vi "assignment - server.vi"() -> ()   [LabVIEW 2020]
panel:
  out "Automation":bool
  out "Vacation":bool
  out "DiningBrightness":u8
  out "KitchenBrightness":u8
  out "Bathroom2Brightness":u8
  out "Bathroom1Brightness":u8
  out "Laundry4Brightness":u8
  out "Laundry3Brightness":u8
  out "Laundry2Brightness":u8
  out "Laundry1Brightness":u8
  out "Bedroom2Brightness":u8
  out "Bedroom1Brightness":u8
  out "LivingRoomBrightness":u8
  out "DayCurtain":bool=TRUE
  out "NightTV":bool=TRUE
  out "Temperature Fluctuations":dbl(graph)
  in  "Upper Temp":dbl
  in  "Lower Temp":dbl
  out "Back Door  Open":bool
  out "Laundry 1 Open":bool
  out "Laundry 2 Open":bool
  out "Bathroom 2 Open":bool
  out "Laundry 4 Open":bool
  out "Bedroom 1 Open":bool
  out "Bedroom 2 Open":bool
  out "Front Door Open":bool
  out "Laundry 4 Close":bool
  out "Laundry 1 Close":bool
  out "Laundry 2 Close":bool
  out "Bathroom 2 Close":bool
  out "Bedroom 2 Close":bool
  out "Bedroom 1 Close":bool
  out "Back Door Close":bool
  out "Front Door Close":bool
  out "Thermometer":dbl(slide) scale=0.0..100.0
  out "Bedroom 2":dbl(slide) scale=0.0..1.0
  out "Bedroom 1":dbl(slide) scale=0.0..1.0
  in  "TV":refnum<k7>(container)
  out "Bathroom 2":bool
  out "Bathroom 1":bool
  out "Laundry 4":bool
  out "Laundry 3":bool
  out "Laundry 2":bool
  out "Laundry 1":bool
  out "Kitchen":bool
  out "Dining":bool
  out "Living Room":bool
  out "Bedroom 2":bool
  out "Bedroom 1":bool
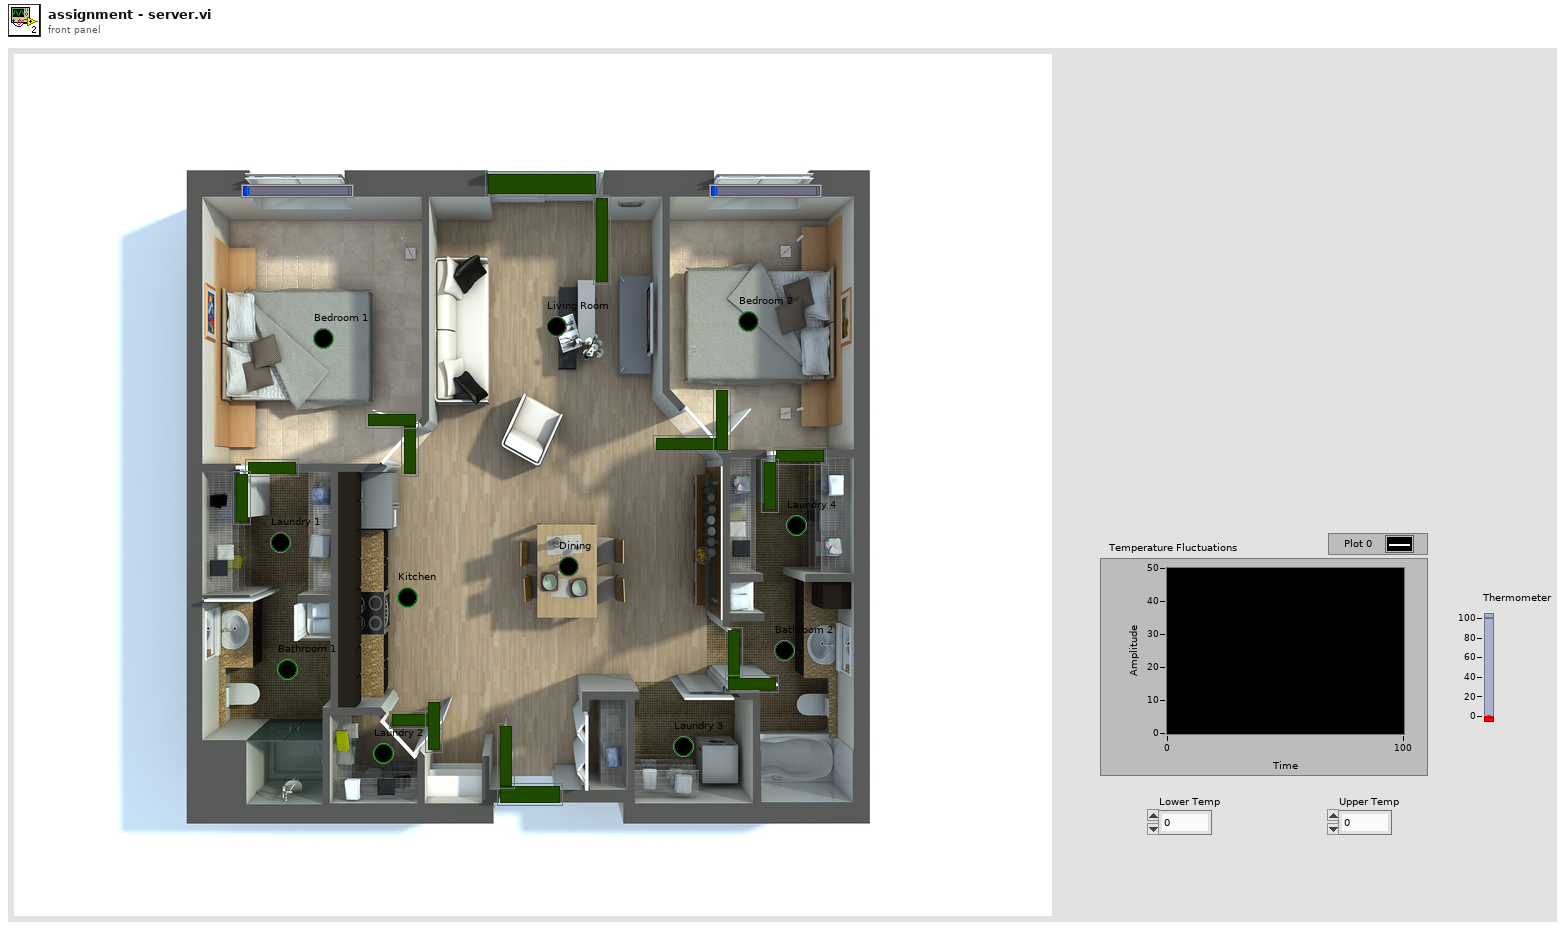
[diagram p1: front panel]
types:
  T1 = typedef "LVDateTimeRec.ctl" = cluster{"fractional second":dbl, "second":i32, "minute":i32, "hour":i32, "day of month":i32, "month":i32, "year":i32, "day of week":i32, "day of year":i32, "DST":i32}
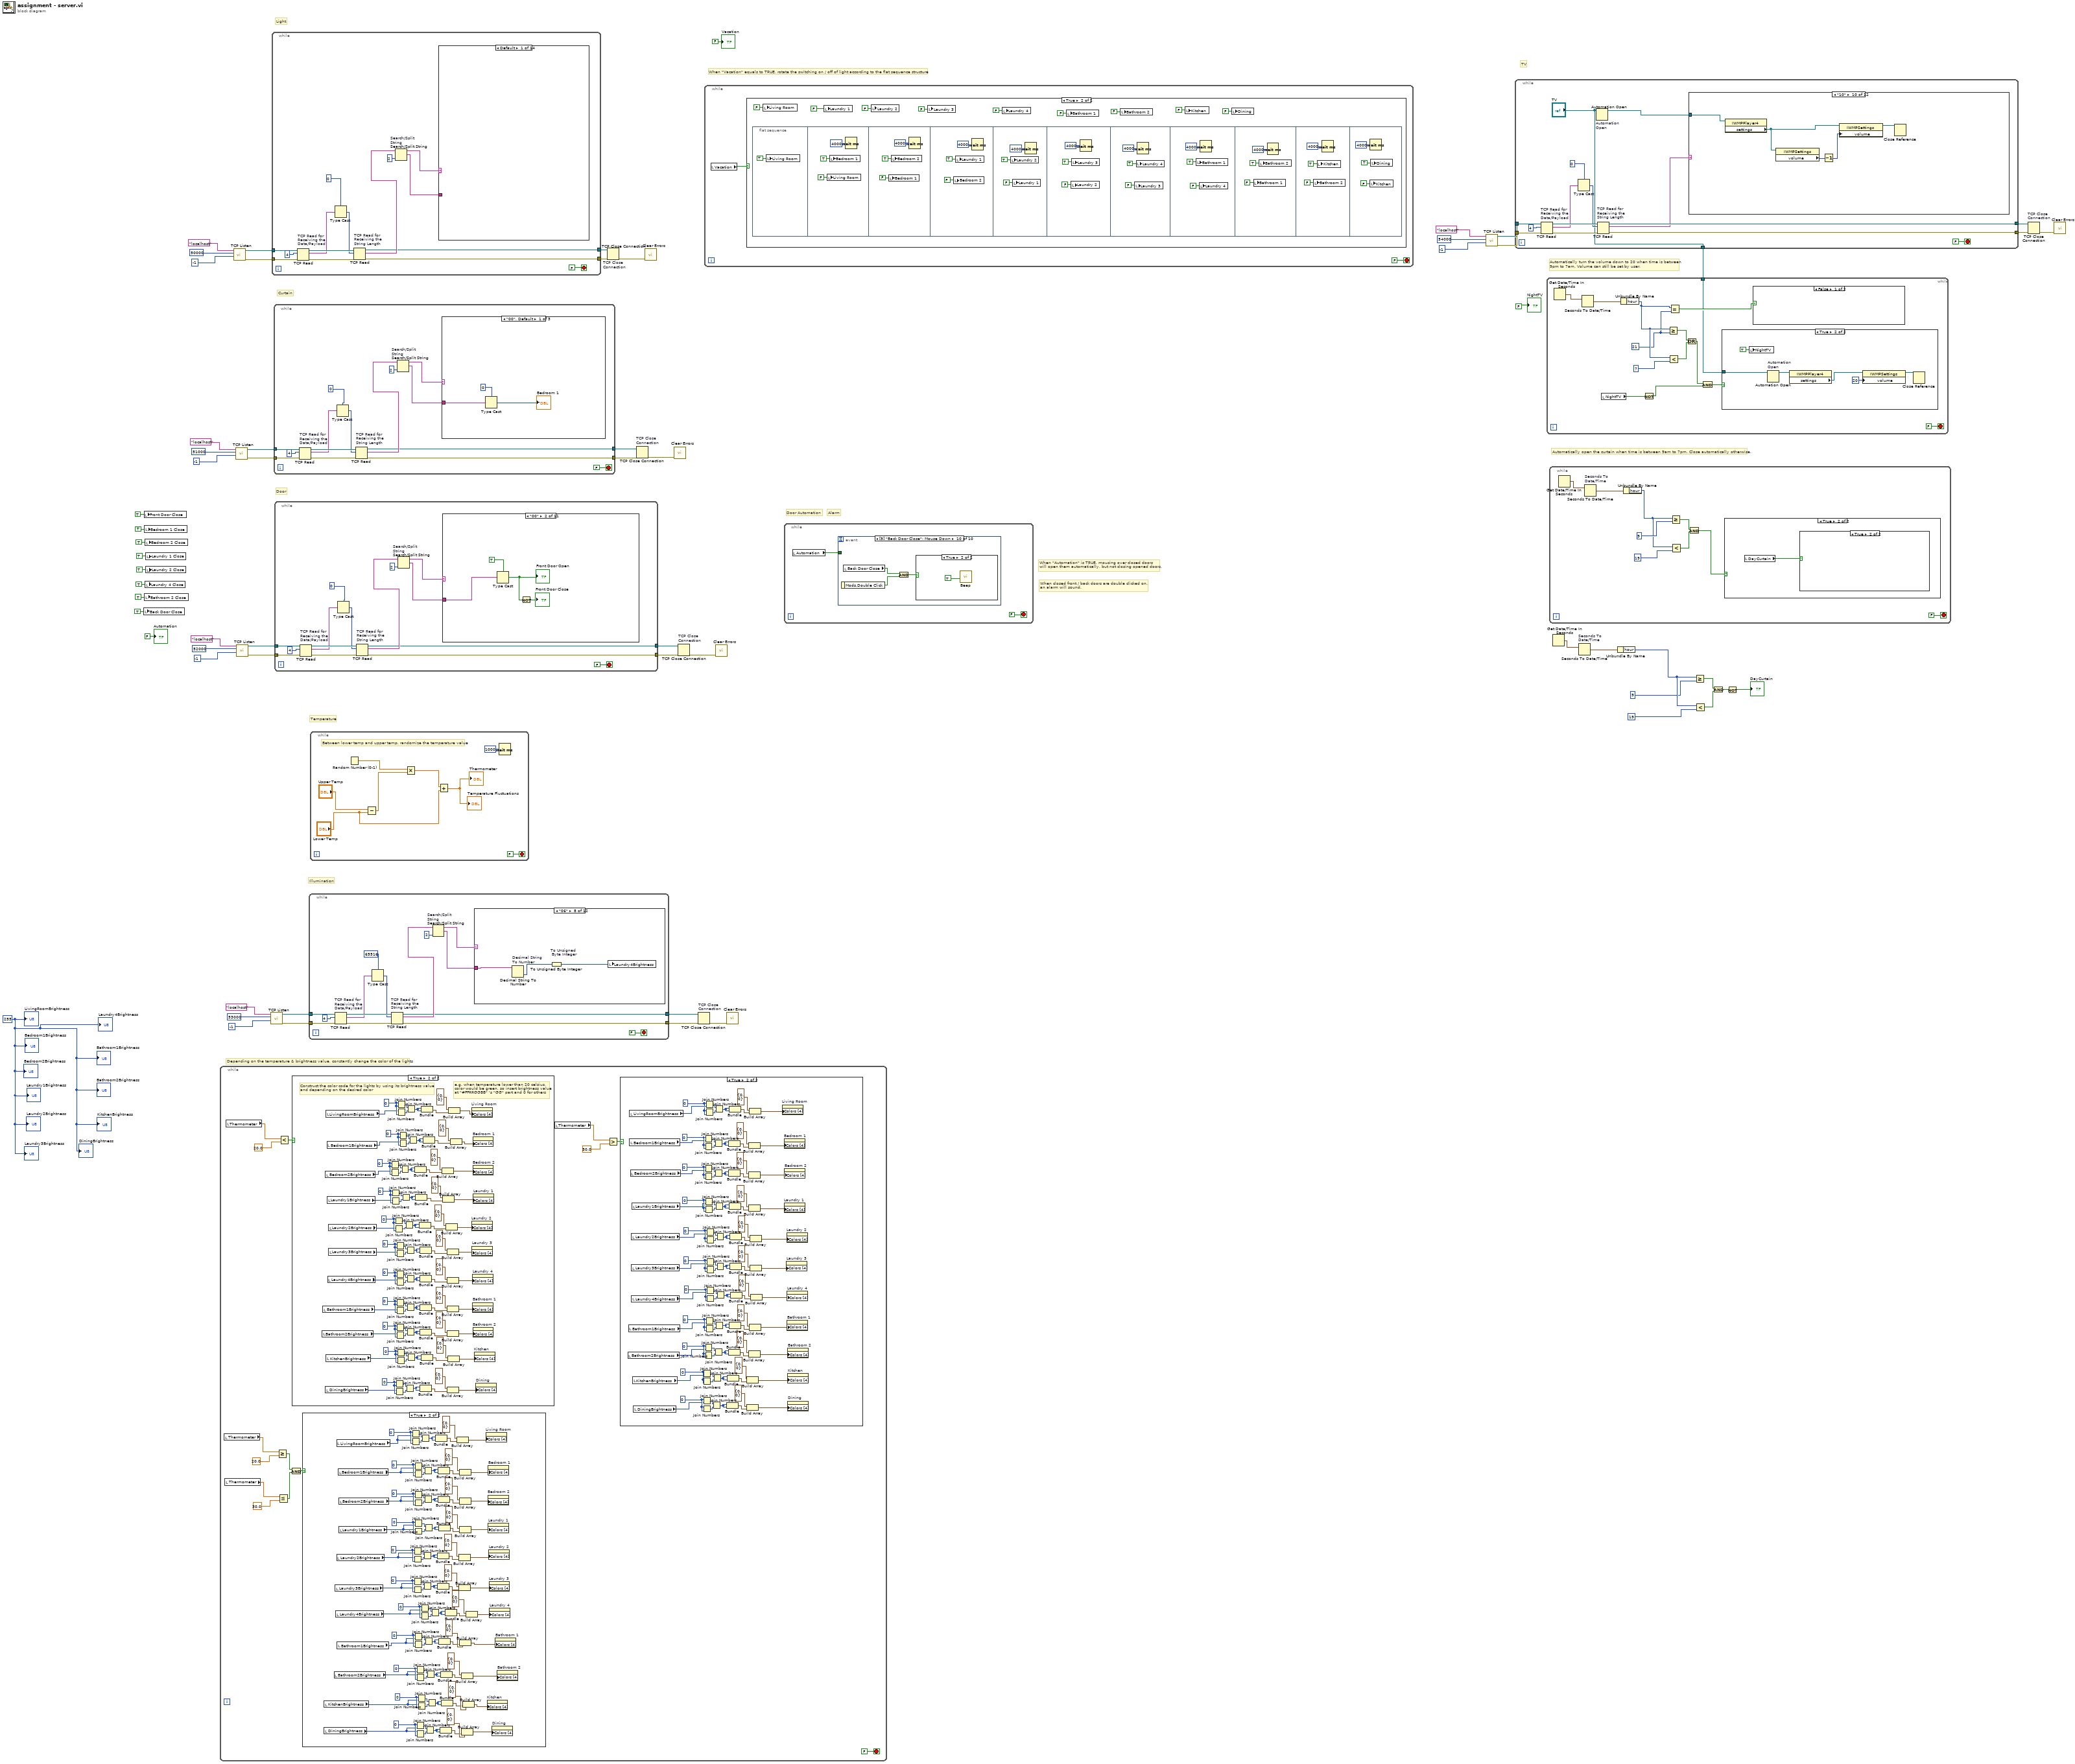
[diagram p0: block diagram]
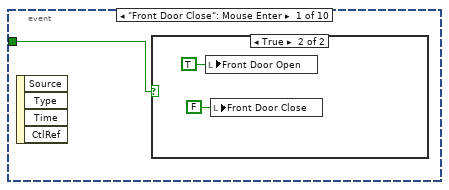
[diagram p2: hidden frame]
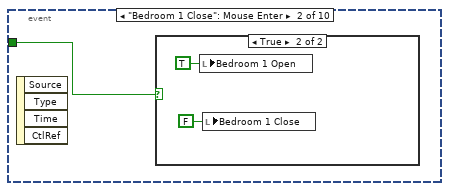
[diagram p4: hidden frame]
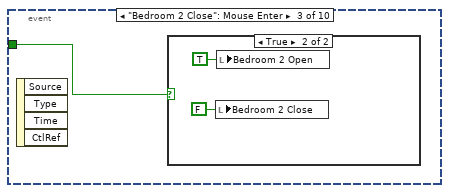
[diagram p6: hidden frame]
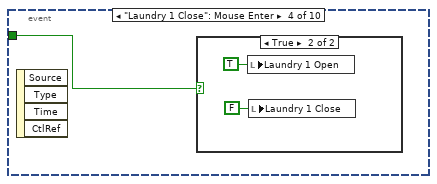
[diagram p8: hidden frame]
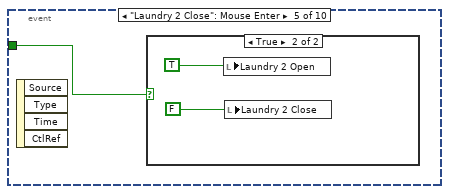
[diagram p10: hidden frame]
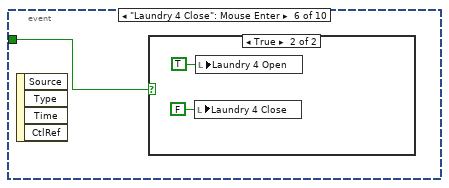
[diagram p12: hidden frame]
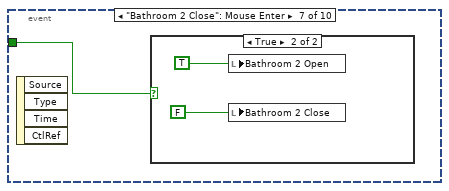
[diagram p14: hidden frame]
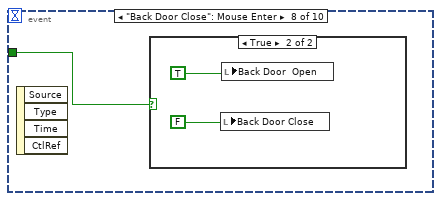
[diagram p16: hidden frame]
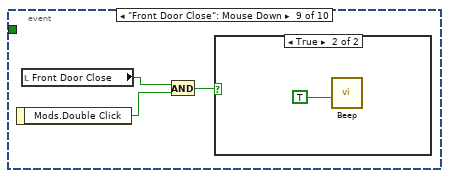
[diagram p18: hidden frame]
diagram:
  w3 = u8 255 ("LivingRoomBrightness")
  # "Automatically open the curtain when time is between 9am to 7pm. Close automatically otherwise."
  # "Automatically turn the volume down to 20 when time is between\n9pm to 7am. Volume can still be set by user."
  # "When \"Vacation\" equals to TRUE, rotate the switching on / off of light according to the flat sequence structure"
  # "When closed front / back doors are double clicked on,\nan alarm will sound."
  # "When \"Automation\" is TRUE, mousing over closed doors\nwill open them automatically, but not closing opened doors."
  # "Depending on the temperature & brightness value, constantly change the color of the lights"
  # "Alarm"
  # "Door Automation"
  # "Illumination"
  # "Temperature"
  # "Door"
  # "Curtain"
  # "TV"
  # "Light"
  n1 = local write "Back Door Close"(TRUE ("Back Door Close")) -> ()
  n2 = local write "Front Door Close"(TRUE ("Front Door Close")) -> ()
  n3 = local write "Bedroom 1 Close"(TRUE ("Bedroom 1 Close")) -> ()
  n4 = local write "Bathroom 2 Close"(TRUE ("Bathroom 2 Close")) -> ()
  n5 = local write "Bedroom 2 Close"(TRUE ("Bedroom 2 Close")) -> ()
  n6 = local write "Laundry 4 Close"(TRUE ("Laundry 4 Close")) -> ()
  n7 = local write "Laundry 1 Close"(TRUE ("Laundry 1 Close")) -> ()
  n8 = local write "Laundry 2 Close"(TRUE ("Laundry 2 Close")) -> ()
  n9 = while {
    stop <- FALSE stop-if-true
    n10 = local read "Thermometer"() -> (w68:dbl)
    n11 = local read "Thermometer"() -> (w65:dbl)
    n12 = local read "Thermometer"() -> (w76:dbl)
    n13 = Greater Or Equal?(x=w68, y=20.0) -> (x >= y?=w66:bool)
    n14 = Less Or Equal?(x=w65, y=30.0) -> (x <= y?=w63:bool)
    n15 = Less?(x=w76, y=20.0) -> (x < y?=w74:bool)
    n16 = And(x=w66, y=w63) -> (x .and. y?=w67:bool)
    n17 = case shown="True" w74 {
      frame False {
      }
      frame True {
        w256 = i8 0 ("hi")
        w264 = i8 0 ("hi")
        w272 = i8 0 ("hi")
        w280 = i8 0 ("hi")
        w288 = i8 0 ("hi")
        w296 = i8 0 ("hi")
        w304 = i8 0 ("hi")
        w312 = i8 0 ("hi")
        w320 = i8 0 ("hi")
        w328 = i8 0 ("hi")
        w335 = i8 0 ("hi")
        # "e.g. when temperature lower than 20 celsius,\ncolor would be green, so insert brightness value\nat \"#FFRRGGBB\" 's \"GG\" part and 0 for others"
        # "Construct the color code for the lights by using its brightness value\nand depending on the desired color"
        n18 = local read "Bathroom2Brightness"() -> (w270:u8)
        n19 = local read "Bathroom1Brightness"() -> (w278:u8)
        n20 = local read "Bedroom2Brightness"() -> (w318:u8)
        n21 = local read "DiningBrightness"() -> (w253:u8)
        n22 = local read "LivingRoomBrightness"() -> (w334:u8)
        n23 = local read "KitchenBrightness"() -> (w262:u8)
        n24 = local read "Bedroom1Brightness"() -> (w325:u8)
        n25 = local read "Laundry1Brightness"() -> (w310:u8)
        n26 = local read "Laundry4Brightness"() -> (w286:u8)
        n27 = local read "Laundry2Brightness"() -> (w302:u8)
        n28 = local read "Laundry3Brightness"() -> (w294:u8)
        n29 = Join Numbers(hi=w320, lo=w320) -> ((hi.lo)=w324:u16)
        n30 = Join Numbers(hi=w318, lo=w320) -> ((hi.lo)=w323:u16)
        n31 = Join Numbers(hi=w312, lo=w312) -> ((hi.lo)=w316:u16)
        n32 = Join Numbers(hi=w310, lo=w312) -> ((hi.lo)=w315:u16)
        n33 = Join Numbers(hi=w304, lo=w304) -> ((hi.lo)=w308:u16)
        n34 = Join Numbers(hi=w302, lo=w304) -> ((hi.lo)=w307:u16)
        n35 = Join Numbers(hi=w256, lo=w256) -> ((hi.lo)=w260:u16)
        n36 = Join Numbers(hi=w253, lo=w256) -> ((hi.lo)=w259:u16)
        n37 = Join Numbers(hi=w296, lo=w296) -> ((hi.lo)=w300:u16)
        n38 = Join Numbers(hi=w294, lo=w296) -> ((hi.lo)=w299:u16)
        n39 = Join Numbers(hi=w288, lo=w288) -> ((hi.lo)=w292:u16)
        n40 = Join Numbers(hi=w286, lo=w288) -> ((hi.lo)=w291:u16)
        n41 = Join Numbers(hi=w280, lo=w280) -> ((hi.lo)=w284:u16)
        n42 = Join Numbers(hi=w278, lo=w280) -> ((hi.lo)=w283:u16)
        n43 = Join Numbers(hi=w272, lo=w272) -> ((hi.lo)=w276:u16)
        n44 = Join Numbers(hi=w270, lo=w272) -> ((hi.lo)=w275:u16)
        n45 = Join Numbers(hi=w264, lo=w264) -> ((hi.lo)=w268:u16)
        n46 = Join Numbers(hi=w262, lo=w264) -> ((hi.lo)=w267:u16)
        n47 = Join Numbers(hi=w335, lo=w335) -> ((hi.lo)=w340:u16)
        n48 = Join Numbers(hi=w334, lo=w335) -> ((hi.lo)=w339:u16)
        n49 = Join Numbers(hi=w328, lo=w328) -> ((hi.lo)=w332:u16)
        n50 = Join Numbers(hi=w325, lo=w328) -> ((hi.lo)=w331:u16)
        n51 = Join Numbers(hi=w324, lo=w323) -> ((hi.lo)=w322:u32)
        n52 = Join Numbers(hi=w316, lo=w315) -> ((hi.lo)=w314:u32)
        n53 = Join Numbers(hi=w308, lo=w307) -> ((hi.lo)=w306:u32)
        n54 = Join Numbers(hi=w260, lo=w259) -> ((hi.lo)=w258:u32)
        n55 = Join Numbers(hi=w300, lo=w299) -> ((hi.lo)=w298:u32)
        n56 = Join Numbers(hi=w292, lo=w291) -> ((hi.lo)=w290:u32)
        n57 = Join Numbers(hi=w284, lo=w283) -> ((hi.lo)=w282:u32)
        n58 = Join Numbers(hi=w276, lo=w275) -> ((hi.lo)=w274:u32)
        n59 = Join Numbers(hi=w268, lo=w267) -> ((hi.lo)=w266:u32)
        n60 = Join Numbers(hi=w340, lo=w339) -> ((hi.lo)=w338:u32)
        n61 = Join Numbers(hi=w332, lo=w331) -> ((hi.lo)=w330:u32)
        n62 = Bundle "Bundle"(w322, w322) -> (w321:cluster{u32, u32})  [unwired: 1 in]
        n63 = Bundle "Bundle"(w314, w314) -> (w313:cluster{u32, u32})  [unwired: 1 in]
        n64 = Bundle "Bundle"(w306, w306) -> (w305:cluster{u32, u32})  [unwired: 1 in]
        n65 = Bundle "Bundle"(w258, w258) -> (w257:cluster{u32, u32})  [unwired: 1 in]
        n66 = Bundle "Bundle"(w298, w298) -> (w297:cluster{u32, u32})  [unwired: 1 in]
        n67 = Bundle "Bundle"(w290, w290) -> (w289:cluster{u32, u32})  [unwired: 1 in]
        n68 = Bundle "Bundle"(w282, w282) -> (w281:cluster{u32, u32})  [unwired: 1 in]
        n69 = Bundle "Bundle"(w274, w274) -> (w273:cluster{u32, u32})  [unwired: 1 in]
        n70 = Bundle "Bundle"(w266, w266) -> (w265:cluster{u32, u32})  [unwired: 1 in]
        n71 = Bundle "Bundle"(w338, w338) -> (w337:cluster{u32, u32})  [unwired: 1 in]
        n72 = Bundle "Bundle"(w330, w330) -> (w329:cluster{u32, u32})  [unwired: 1 in]
        n73 = Build Array "Build Array"(cluster{u32, u32} {0, 0} ("element"), w321) -> (w317:cluster{u32, u32}[])
        n74 = Build Array "Build Array"(cluster{u32, u32} {0, 0} ("element"), w313) -> (w309:cluster{u32, u32}[])
        n75 = Build Array "Build Array"(cluster{u32, u32} {0, 0} ("element"), w305) -> (w301:cluster{u32, u32}[])
        n76 = Build Array "Build Array"(cluster{u32, u32} {0, 0} ("element"), w257) -> (w254:cluster{u32, u32}[])
        n77 = Build Array "Build Array"(cluster{u32, u32} {0, 0} ("element"), w297) -> (w293:cluster{u32, u32}[])
        n78 = Build Array "Build Array"(cluster{u32, u32} {0, 0} ("element"), w289) -> (w285:cluster{u32, u32}[])
        n79 = Build Array "Build Array"(cluster{u32, u32} {0, 0} ("element"), w281) -> (w277:cluster{u32, u32}[])
        n80 = Build Array "Build Array"(cluster{u32, u32} {0, 0} ("element"), w273) -> (w269:cluster{u32, u32}[])
        n81 = Build Array "Build Array"(cluster{u32, u32} {0, 0} ("element"), w265) -> (w261:cluster{u32, u32}[])
        n82 = Build Array "Build Array"(cluster{u32, u32} {0, 0} ("element"), w337) -> (w336:cluster{u32, u32}[])
        n83 = Build Array "Build Array"(cluster{u32, u32} {0, 0} ("element"), w329) -> (w326:cluster{u32, u32}[])
        n84 = property on="Living Room" class="Bool (strict)"("Colors [4]"=w336) -> ()  [unwired: 2 in, 2 out]
        n85 = property on="Laundry 2" class="Bool (strict)"("Colors [4]"=w301) -> ()  [unwired: 2 in, 2 out]
        n86 = property on="Laundry 3" class="Bool (strict)"("Colors [4]"=w293) -> ()  [unwired: 2 in, 2 out]
        n87 = property on="Laundry 4" class="Bool (strict)"("Colors [4]"=w285) -> ()  [unwired: 2 in, 2 out]
        n88 = property on="Bathroom 1" class="Bool (strict)"("Colors [4]"=w277) -> ()  [unwired: 2 in, 2 out]
        n89 = property on="Bedroom 1" class="Bool (strict)"("Colors [4]"=w326) -> ()  [unwired: 2 in, 2 out]
        n90 = property on="Bedroom 2" class="Bool (strict)"("Colors [4]"=w317) -> ()  [unwired: 2 in, 2 out]
        n91 = property on="Bathroom 2" class="Bool (strict)"("Colors [4]"=w269) -> ()  [unwired: 2 in, 2 out]
        n92 = property on="Laundry 1" class="Bool (strict)"("Colors [4]"=w309) -> ()  [unwired: 2 in, 2 out]
        n93 = property on="Kitchen" class="Bool (strict)"("Colors [4]"=w261) -> ()  [unwired: 2 in, 2 out]
        n94 = property on="Dining" class="Bool (strict)"("Colors [4]"=w254) -> ()  [unwired: 2 in, 2 out]
      }
    }
    n95 = case shown="True" w67 {
      frame False {
      }
      frame True {
        w82 = i8 0 ("hi")
        w90 = i8 0 ("hi")
        w98 = i8 0 ("hi")
        w106 = i8 0 ("hi")
        w114 = i8 0 ("hi")
        w122 = i8 0 ("hi")
        w130 = i8 0 ("hi")
        w138 = i8 0 ("hi")
        w146 = i8 0 ("hi")
        w154 = i8 0 ("hi")
        w161 = i8 0 ("hi")
        n96 = local read "KitchenBrightness"() -> (w86:u8)
        n97 = local read "DiningBrightness"() -> (w78:u8)
        n98 = local read "Bathroom2Brightness"() -> (w94:u8)
        n99 = local read "Laundry3Brightness"() -> (w118:u8)
        n100 = local read "Laundry4Brightness"() -> (w110:u8)
        n101 = local read "LivingRoomBrightness"() -> (w160:u8)
        n102 = local read "Laundry2Brightness"() -> (w126:u8)
        n103 = local read "Bathroom1Brightness"() -> (w102:u8)
        n104 = local read "Bedroom1Brightness"() -> (w150:u8)
        n105 = local read "Bedroom2Brightness"() -> (w142:u8)
        n106 = local read "Laundry1Brightness"() -> (w134:u8)
        n107 = Join Numbers(hi=w161, lo=w160) -> ((hi.lo)=w162:u16)
        n108 = Join Numbers(hi=w160, lo=w161) -> ((hi.lo)=w163:u16)
        n109 = Join Numbers(hi=w130, lo=w126) -> ((hi.lo)=w129:u16)
        n110 = Join Numbers(hi=w126, lo=w130) -> ((hi.lo)=w128:u16)
        n111 = Join Numbers(hi=w122, lo=w118) -> ((hi.lo)=w121:u16)
        n112 = Join Numbers(hi=w118, lo=w122) -> ((hi.lo)=w120:u16)
        n113 = Join Numbers(hi=w154, lo=w150) -> ((hi.lo)=w153:u16)
        n114 = Join Numbers(hi=w150, lo=w154) -> ((hi.lo)=w152:u16)
        n115 = Join Numbers(hi=w146, lo=w142) -> ((hi.lo)=w145:u16)
        n116 = Join Numbers(hi=w142, lo=w146) -> ((hi.lo)=w144:u16)
        n117 = Join Numbers(hi=w138, lo=w134) -> ((hi.lo)=w137:u16)
        n118 = Join Numbers(hi=w134, lo=w138) -> ((hi.lo)=w136:u16)
        n119 = Join Numbers(hi=w106, lo=w102) -> ((hi.lo)=w105:u16)
        n120 = Join Numbers(hi=w102, lo=w106) -> ((hi.lo)=w104:u16)
        n121 = Join Numbers(hi=w82, lo=w78) -> ((hi.lo)=w81:u16)
        n122 = Join Numbers(hi=w78, lo=w82) -> ((hi.lo)=w80:u16)
        n123 = Join Numbers(hi=w98, lo=w94) -> ((hi.lo)=w97:u16)
        n124 = Join Numbers(hi=w94, lo=w98) -> ((hi.lo)=w96:u16)
        n125 = Join Numbers(hi=w90, lo=w86) -> ((hi.lo)=w89:u16)
        n126 = Join Numbers(hi=w86, lo=w90) -> ((hi.lo)=w88:u16)
        n127 = Join Numbers(hi=w114, lo=w110) -> ((hi.lo)=w113:u16)
        n128 = Join Numbers(hi=w110, lo=w114) -> ((hi.lo)=w112:u16)
        n129 = Join Numbers(hi=w162, lo=w163) -> ((hi.lo)=w164:u32)
        n130 = Join Numbers(hi=w129, lo=w128) -> ((hi.lo)=w127:u32)
        n131 = Join Numbers(hi=w121, lo=w120) -> ((hi.lo)=w119:u32)
        n132 = Join Numbers(hi=w153, lo=w152) -> ((hi.lo)=w151:u32)
        n133 = Join Numbers(hi=w145, lo=w144) -> ((hi.lo)=w143:u32)
        n134 = Join Numbers(hi=w137, lo=w136) -> ((hi.lo)=w135:u32)
        n135 = Join Numbers(hi=w105, lo=w104) -> ((hi.lo)=w103:u32)
        n136 = Join Numbers(hi=w81, lo=w80) -> ((hi.lo)=w79:u32)
        n137 = Join Numbers(hi=w97, lo=w96) -> ((hi.lo)=w95:u32)
        n138 = Join Numbers(hi=w89, lo=w88) -> ((hi.lo)=w87:u32)
        n139 = Join Numbers(hi=w113, lo=w112) -> ((hi.lo)=w111:u32)
        n140 = Bundle(w164, w164) -> (w159:cluster{u32, u32})  [unwired: 1 in]
        n141 = Bundle(w127, w127) -> (w131:cluster{u32, u32})  [unwired: 1 in]
        n142 = Bundle(w119, w119) -> (w123:cluster{u32, u32})  [unwired: 1 in]
        n143 = Bundle(w151, w151) -> (w155:cluster{u32, u32})  [unwired: 1 in]
        n144 = Bundle(w143, w143) -> (w147:cluster{u32, u32})  [unwired: 1 in]
        n145 = Bundle(w135, w135) -> (w139:cluster{u32, u32})  [unwired: 1 in]
        n146 = Bundle(w103, w103) -> (w107:cluster{u32, u32})  [unwired: 1 in]
        n147 = Bundle(w79, w79) -> (w83:cluster{u32, u32})  [unwired: 1 in]
        n148 = Bundle(w95, w95) -> (w99:cluster{u32, u32})  [unwired: 1 in]
        n149 = Bundle(w87, w87) -> (w91:cluster{u32, u32})  [unwired: 1 in]
        n150 = Bundle(w111, w111) -> (w115:cluster{u32, u32})  [unwired: 1 in]
        n151 = Build Array "Build Array"(cluster{u32, u32} {0, 0} ("element"), w159) -> (w157:cluster{u32, u32}[])
        n152 = Build Array "Build Array"(cluster{u32, u32} {0, 0} ("element"), w131) -> (w125:cluster{u32, u32}[])
        n153 = Build Array "Build Array"(cluster{u32, u32} {0, 0} ("element"), w123) -> (w117:cluster{u32, u32}[])
        n154 = Build Array "Build Array"(cluster{u32, u32} {0, 0} ("element"), w155) -> (w149:cluster{u32, u32}[])
        n155 = Build Array "Build Array"(cluster{u32, u32} {0, 0} ("element"), w147) -> (w141:cluster{u32, u32}[])
        n156 = Build Array "Build Array"(cluster{u32, u32} {0, 0} ("element"), w139) -> (w133:cluster{u32, u32}[])
        n157 = Build Array "Build Array"(cluster{u32, u32} {0, 0} ("element"), w107) -> (w101:cluster{u32, u32}[])
        n158 = Build Array "Build Array"(cluster{u32, u32} {0, 0} ("element"), w83) -> (w77:cluster{u32, u32}[])
        n159 = Build Array "Build Array"(cluster{u32, u32} {0, 0} ("element"), w99) -> (w93:cluster{u32, u32}[])
        n160 = Build Array "Build Array"(cluster{u32, u32} {0, 0} ("element"), w91) -> (w85:cluster{u32, u32}[])
        n161 = Build Array "Build Array"(cluster{u32, u32} {0, 0} ("element"), w115) -> (w109:cluster{u32, u32}[])
        n162 = property on="Living Room" class="Bool (strict)"("Colors [4]"=w157) -> ()  [unwired: 2 in, 2 out]
        n163 = property on="Kitchen" class="Bool (strict)"("Colors [4]"=w85) -> ()  [unwired: 2 in, 2 out]
        n164 = property on="Bedroom 2" class="Bool (strict)"("Colors [4]"=w141) -> ()  [unwired: 2 in, 2 out]
        n165 = property on="Bedroom 1" class="Bool (strict)"("Colors [4]"=w149) -> ()  [unwired: 2 in, 2 out]
        n166 = property on="Laundry 1" class="Bool (strict)"("Colors [4]"=w133) -> ()  [unwired: 2 in, 2 out]
        n167 = property on="Laundry 2" class="Bool (strict)"("Colors [4]"=w125) -> ()  [unwired: 2 in, 2 out]
        n168 = property on="Laundry 3" class="Bool (strict)"("Colors [4]"=w117) -> ()  [unwired: 2 in, 2 out]
        n169 = property on="Laundry 4" class="Bool (strict)"("Colors [4]"=w109) -> ()  [unwired: 2 in, 2 out]
        n170 = property on="Dining" class="Bool (strict)"("Colors [4]"=w77) -> ()  [unwired: 2 in, 2 out]
        n171 = property on="Bathroom 1" class="Bool (strict)"("Colors [4]"=w101) -> ()  [unwired: 2 in, 2 out]
        n172 = property on="Bathroom 2" class="Bool (strict)"("Colors [4]"=w93) -> ()  [unwired: 2 in, 2 out]
      }
    }
    n173 = local read "Thermometer"() -> (w70:dbl)
    n174 = Greater?(x=w70, y=30.0) -> (0:w72:bool)
    n175 = case shown="True" w72 {
      frame False {
      }
      frame True {
        w169 = i8 0 ("hi")
        w176 = i8 0 ("hi")
        w185 = i8 0 ("hi")
        w193 = i8 0 ("hi")
        w201 = i8 0 ("hi")
        w209 = i8 0 ("hi")
        w216 = i8 0 ("hi")
        w225 = i8 0 ("hi")
        w233 = i8 0 ("hi")
        w241 = i8 0 ("hi")
        w248 = i8 0 ("hi")
        n176 = local read "Bathroom2Brightness"() -> (w182:u8)
        n177 = local read "Bathroom1Brightness"() -> (w190:u8)
        n178 = local read "LivingRoomBrightness"() -> (w249:u8)
        n179 = local read "Bedroom1Brightness"() -> (w237:u8)
        n180 = local read "Bedroom2Brightness"() -> (w229:u8)
        n181 = local read "Laundry2Brightness"() -> (w214:u8)
        n182 = local read "Laundry3Brightness"() -> (w206:u8)
        n183 = local read "Laundry4Brightness"() -> (w198:u8)
        n184 = local read "Laundry1Brightness"() -> (w222:u8)
        n185 = local read "KitchenBrightness"() -> (w173:u8)
        n186 = local read "DiningBrightness"() -> (w166:u8)
        n187 = Join Numbers(hi=w169, lo=w166) -> ((hi.lo)=w170:u16)
        n188 = Join Numbers(hi=w169, lo=w169) -> ((hi.lo)=w171:u16)
        n189 = Join Numbers(hi=w176, lo=w173) -> ((hi.lo)=w179:u16)
        n190 = Join Numbers(hi=w176, lo=w176) -> ((hi.lo)=w178:u16)
        n191 = Join Numbers(hi=w241, lo=w237) -> ((hi.lo)=w242:u16)
        n192 = Join Numbers(hi=w241, lo=w241) -> ((hi.lo)=w243:u16)
        n193 = Join Numbers(hi=w233, lo=w229) -> ((hi.lo)=w234:u16)
        n194 = Join Numbers(hi=w233, lo=w233) -> ((hi.lo)=w235:u16)
        n195 = Join Numbers(hi=w185, lo=w182) -> ((hi.lo)=w186:u16)
        n196 = Join Numbers(hi=w185, lo=w185) -> ((hi.lo)=w187:u16)
        n197 = Join Numbers(hi=w225, lo=w222) -> ((hi.lo)=w226:u16)
        n198 = Join Numbers(hi=w225, lo=w225) -> ((hi.lo)=w227:u16)
        n199 = Join Numbers(hi=w248, lo=w249) -> ((hi.lo)=w250:u16)
        n200 = Join Numbers(hi=w248, lo=w248) -> ((hi.lo)=w251:u16)
        n201 = Join Numbers(hi=w193, lo=w190) -> ((hi.lo)=w194:u16)
        n202 = Join Numbers(hi=w193, lo=w193) -> ((hi.lo)=w195:u16)
        n203 = Join Numbers(hi=w216, lo=w214) -> ((hi.lo)=w219:u16)
        n204 = Join Numbers(hi=w216, lo=w216) -> ((hi.lo)=w218:u16)
        n205 = Join Numbers(hi=w209, lo=w206) -> ((hi.lo)=w210:u16)
        n206 = Join Numbers(hi=w209, lo=w209) -> ((hi.lo)=w211:u16)
        n207 = Join Numbers(hi=w201, lo=w198) -> ((hi.lo)=w202:u16)
        n208 = Join Numbers(hi=w201, lo=w201) -> ((hi.lo)=w203:u16)
        n209 = Join Numbers(hi=w170, lo=w171) -> ((hi.lo)=w172:u32)
        n210 = Join Numbers(hi=w179, lo=w178) -> ((hi.lo)=w177:u32)
        n211 = Join Numbers(hi=w242, lo=w243) -> ((hi.lo)=w244:u32)
        n212 = Join Numbers(hi=w234, lo=w235) -> ((hi.lo)=w236:u32)
        n213 = Join Numbers(hi=w186, lo=w187) -> ((hi.lo)=w188:u32)
        n214 = Join Numbers(hi=w226, lo=w227) -> ((hi.lo)=w228:u32)
        n215 = Join Numbers(hi=w250, lo=w251) -> ((hi.lo)=w252:u32)
        n216 = Join Numbers(hi=w194, lo=w195) -> ((hi.lo)=w196:u32)
        n217 = Join Numbers(hi=w219, lo=w218) -> ((hi.lo)=w217:u32)
        n218 = Join Numbers(hi=w210, lo=w211) -> ((hi.lo)=w212:u32)
        n219 = Join Numbers(hi=w202, lo=w203) -> ((hi.lo)=w204:u32)
        n220 = Bundle(w172, w172) -> (w168:cluster{u32, u32})  [unwired: 1 in]
        n221 = Bundle(w177, w177) -> (w180:cluster{u32, u32})  [unwired: 1 in]
        n222 = Bundle(w244, w244) -> (w240:cluster{u32, u32})  [unwired: 1 in]
        n223 = Bundle(w236, w236) -> (w232:cluster{u32, u32})  [unwired: 1 in]
        n224 = Bundle(w188, w188) -> (w184:cluster{u32, u32})  [unwired: 1 in]
        n225 = Bundle(w228, w228) -> (w224:cluster{u32, u32})  [unwired: 1 in]
        n226 = Bundle(w252, w252) -> (w247:cluster{u32, u32})  [unwired: 1 in]
        n227 = Bundle(w196, w196) -> (w192:cluster{u32, u32})  [unwired: 1 in]
        n228 = Bundle(w217, w217) -> (w220:cluster{u32, u32})  [unwired: 1 in]
        n229 = Bundle(w212, w212) -> (w208:cluster{u32, u32})  [unwired: 1 in]
        n230 = Bundle(w204, w204) -> (w200:cluster{u32, u32})  [unwired: 1 in]
        n231 = Build Array "Build Array"(cluster{u32, u32} {0, 0} ("element"), w168) -> (w165:cluster{u32, u32}[])
        n232 = Build Array "Build Array"(cluster{u32, u32} {0, 0} ("element"), w180) -> (w174:cluster{u32, u32}[])
        n233 = Build Array "Build Array"(cluster{u32, u32} {0, 0} ("element"), w240) -> (w238:cluster{u32, u32}[])
        n234 = Build Array "Build Array"(cluster{u32, u32} {0, 0} ("element"), w232) -> (w230:cluster{u32, u32}[])
        n235 = Build Array "Build Array"(cluster{u32, u32} {0, 0} ("element"), w184) -> (w181:cluster{u32, u32}[])
        n236 = Build Array "Build Array"(cluster{u32, u32} {0, 0} ("element"), w224) -> (w221:cluster{u32, u32}[])
        n237 = Build Array "Build Array"(cluster{u32, u32} {0, 0} ("element"), w247) -> (w245:cluster{u32, u32}[])
        n238 = Build Array "Build Array"(cluster{u32, u32} {0, 0} ("element"), w192) -> (w189:cluster{u32, u32}[])
        n239 = Build Array "Build Array"(cluster{u32, u32} {0, 0} ("element"), w220) -> (w213:cluster{u32, u32}[])
        n240 = Build Array "Build Array"(cluster{u32, u32} {0, 0} ("element"), w208) -> (w205:cluster{u32, u32}[])
        n241 = Build Array "Build Array"(cluster{u32, u32} {0, 0} ("element"), w200) -> (w197:cluster{u32, u32}[])
        n242 = property on="Living Room" class="Bool (strict)"("Colors [4]"=w245) -> ()  [unwired: 2 in, 2 out]
        n243 = property on="Bedroom 1" class="Bool (strict)"("Colors [4]"=w238) -> ()  [unwired: 2 in, 2 out]
        n244 = property on="Laundry 1" class="Bool (strict)"("Colors [4]"=w221) -> ()  [unwired: 2 in, 2 out]
        n245 = property on="Bedroom 2" class="Bool (strict)"("Colors [4]"=w230) -> ()  [unwired: 2 in, 2 out]
        n246 = property on="Laundry 3" class="Bool (strict)"("Colors [4]"=w205) -> ()  [unwired: 2 in, 2 out]
        n247 = property on="Laundry 2" class="Bool (strict)"("Colors [4]"=w213) -> ()  [unwired: 2 in, 2 out]
        n248 = property on="Laundry 4" class="Bool (strict)"("Colors [4]"=w197) -> ()  [unwired: 2 in, 2 out]
        n249 = property on="Bathroom 1" class="Bool (strict)"("Colors [4]"=w189) -> ()  [unwired: 2 in, 2 out]
        n250 = property on="Bathroom 2" class="Bool (strict)"("Colors [4]"=w181) -> ()  [unwired: 2 in, 2 out]
        n251 = property on="Kitchen" class="Bool (strict)"("Colors [4]"=w174) -> ()  [unwired: 2 in, 2 out]
        n252 = property on="Dining" class="Bool (strict)"("Colors [4]"=w165) -> ()  [unwired: 2 in, 2 out]
      }
    }
  }
  n253 = call <vilib>:"TCP Listen.vi"("timeout ms (wait forever: -1)"=-1, "port"=u16 50000, "service name"="localhost") -> ("error out"=w58:errorcluster, "connection ID"=w59:refnum<k5>)  [unwired: 4 in, 3 out]
  n254 = call <vilib>:"TCP Listen.vi"("timeout ms (wait forever: -1)"=-1, "port"=u16 51000, "service name"="localhost") -> ("error out"=w42:errorcluster, "connection ID"=w43:refnum<k5>)  [unwired: 4 in, 3 out]
  n255 = call <vilib>:"TCP Listen.vi"("timeout ms (wait forever: -1)"=-1, "port"=u16 52000, "service name"="localhost") -> ("error out"=w34:errorcluster, "connection ID"=w35:refnum<k5>)  [unwired: 4 in, 3 out]
  n256 = call <vilib>:"TCP Listen.vi"("timeout ms (wait forever: -1)"=-1, "port"=u16 53000, "service name"="localhost") -> ("error out"=w16:errorcluster, "connection ID"=w17:refnum<k5>)  [unwired: 4 in, 3 out]
  n257 = while {
    tunnel: w59 -> [w355]
    tunnel: w58 -> [w354]
    tunnel: [w346] -> w57
    tunnel: [w345] -> w56
    stop <- FALSE stop-if-true
    n258 = TCP Read "TCP Read for\nReceiving the\nData/Payload"(connection ID=w355, bytes to read=4, error in (no error)=w354) -> (connection ID out=w353:refnum<k5>, data out=w343:string, error out=w352:errorcluster)  [unwired: 2 in]
    n259 = Type Cast(type=0, x=w343) -> (*(type *) &x=w342:i32)
    n260 = TCP Read "TCP Read for\nReceiving the\nString Length"(connection ID=w353, bytes to read=w342, error in (no error)=w352) -> (connection ID out=w346:refnum<k5>, data out=w350:string, error out=w345:errorcluster)  [unwired: 2 in]
    n261 = Search/Split String "Search/Split \nString"(string=w350, offset (0)=2) -> (substring before match=w348:string, match + rest of string=w347:string)  [unwired: 1 in, 1 out]
    n262 = case shown="Default" w348 {
      tunnel: w347 -> [_ w358 w361 w364 w367 w370 w373 w376 w379 w382 w385 w388 w391 w394]
      frame Default {
      }
      frame "00" {
        n263 = Type Cast(type=TRUE, x=w358) -> (*(type *) &x=→"Living Room":bool)
      }
      frame "01" {
        n264 = Type Cast(type=TRUE, x=w361) -> (*(type *) &x=→"Bedroom 1":bool)
      }
      frame "02" {
        n265 = Type Cast(type=TRUE, x=w364) -> (*(type *) &x=→"Bedroom 2":bool)
      }
      frame "03" {
        n266 = Type Cast(type=TRUE, x=w367) -> (*(type *) &x=→"Laundry 1":bool)
      }
      frame "04" {
        n267 = Type Cast(type=TRUE, x=w370) -> (*(type *) &x=→"Laundry 2":bool)
      }
      frame "05" {
        n268 = Type Cast(type=TRUE, x=w373) -> (*(type *) &x=→"Laundry 3":bool)
      }
      frame "06" {
        n269 = Type Cast(type=TRUE, x=w376) -> (*(type *) &x=→"Laundry 4":bool)
      }
      frame "07" {
        n270 = Type Cast(type=TRUE, x=w379) -> (*(type *) &x=→"Bathroom 1":bool)
      }
      frame "08" {
        n271 = Type Cast(type=TRUE, x=w382) -> (*(type *) &x=→"Bathroom 2":bool)
      }
      frame "09" {
        n272 = Type Cast(type=TRUE, x=w385) -> (*(type *) &x=→"Kitchen":bool)
      }
      frame "10" {
        n273 = Type Cast(type=TRUE, x=w388) -> (*(type *) &x=→"Dining":bool)
      }
      frame "11" {
        n274 = Type Cast(type=TRUE, x=w391) -> (*(type *) &x=w389:bool)
        n275 = local write "Living Room"(w389) -> ()
        n276 = local write "Bedroom 2"(w389) -> ()
        n277 = local write "Bathroom 1"(w389) -> ()
        n278 = local write "Bathroom 2"(w389) -> ()
        n279 = local write "Bedroom 1"(w389) -> ()
        n280 = local write "Laundry 3"(w389) -> ()
        n281 = local write "Laundry 4"(w389) -> ()
        n282 = local write "Laundry 1"(w389) -> ()
        n283 = local write "Laundry 2"(w389) -> ()
        n284 = local write "Dining"(w389) -> ()
        n285 = local write "Kitchen"(w389) -> ()
      }
      frame "12" {
        n286 = Type Cast(type=TRUE, x=w394) -> (*(type *) &x=w392:bool)
        n287 = case shown="True" w392 {
          frame True {
            n288 = local write "Vacation"(TRUE ("Vacation")) -> ()
          }
          frame False {
            n289 = local write "Vacation"(FALSE) -> ()
          }
        }
      }
    }
  }
  n290 = while {
    tunnel: w43 -> [w411]
    tunnel: w42 -> [w410]
    tunnel: [w402] -> w41
    tunnel: [w401] -> w40
    stop <- FALSE stop-if-true
    n291 = TCP Read "TCP Read for\nReceiving the\nData/Payload"(connection ID=w411, bytes to read=4, error in (no error)=w410) -> (connection ID out=w409:refnum<k5>, data out=w399:string, error out=w408:errorcluster)  [unwired: 2 in]
    n292 = Type Cast(type=0, x=w399) -> (*(type *) &x=w398:i32)
    n293 = TCP Read "TCP Read for\nReceiving the\nString Length"(connection ID=w409, bytes to read=w398, error in (no error)=w408) -> (connection ID out=w402:refnum<k5>, data out=w406:string, error out=w401:errorcluster)  [unwired: 2 in]
    n294 = Search/Split String "Search/Split \nString"(string=w406, offset (0)=2) -> (substring before match=w404:string, match + rest of string=w403:string)  [unwired: 1 in, 1 out]
    n295 = case shown="\"00\", Default" w404 {
      tunnel: w403 -> [w414 w417 w420]
      frame "00", Default {
        n296 = Type Cast(type=0, x=w414) -> (*(type *) &x=→"Bedroom 1":i32)
      }
      frame "01" {
        n297 = Type Cast(type=0, x=w417) -> (*(type *) &x=→"Bedroom 2":i32)
      }
      frame "02" {
        n298 = Type Cast(type=0, x=w420) -> (*(type *) &x=w418:i32)
        n299 = local write "Bedroom 2"(w418) -> ()
        n300 = local write "Bedroom 1"(w418) -> ()
      }
    }
  }
  n301 = while {
    tunnel: w35 -> [w435]
    tunnel: w34 -> [w434]
    tunnel: [w426] -> w33
    tunnel: [w425] -> w32
    stop <- FALSE stop-if-true
    n302 = TCP Read "TCP Read for\nReceiving the\nData/Payload"(connection ID=w435, bytes to read=4, error in (no error)=w434) -> (connection ID out=w433:refnum<k5>, data out=w423:string, error out=w432:errorcluster)  [unwired: 2 in]
    n303 = Type Cast(type=0, x=w423) -> (*(type *) &x=w422:i32)
    n304 = TCP Read "TCP Read for\nReceiving the\nString Length"(connection ID=w433, bytes to read=w422, error in (no error)=w432) -> (connection ID out=w426:refnum<k5>, data out=w430:string, error out=w425:errorcluster)  [unwired: 2 in]
    n305 = Search/Split String "Search/Split \nString"(string=w430, offset (0)=2) -> (substring before match=w428:string, match + rest of string=w427:string)  [unwired: 1 in, 1 out]
    n306 = case shown="\"00\"" w428 {
      tunnel: w427 -> [_ w439 w443 w447 w451 w455 w459 w463 w467 w471 w474]
      frame Default {
      }
      frame "00" {
        n307 = Type Cast(type=TRUE, x=w439) -> (*(type *) &x=w437:bool)
        "Front Door Open" <- w437
        n308 = Not(x=w437) -> (.not. x?=→"Front Door Close":bool)
      }
      frame "01" {
        n309 = Type Cast(type=TRUE, x=w443) -> (*(type *) &x=w440:bool)
        "Bedroom 1 Open" <- w440
        n310 = Not(x=w440) -> (.not. x?=→"Bedroom 1 Close":bool)
      }
      frame "02" {
        n311 = Type Cast(type=TRUE, x=w447) -> (*(type *) &x=w445:bool)
        "Bedroom 2 Open" <- w445
        n312 = Not(x=w445) -> (.not. x?=→"Bedroom 2 Close":bool)
      }
      frame "03" {
        n313 = Type Cast(type=TRUE, x=w451) -> (*(type *) &x=w449:bool)
        "Laundry 1 Open" <- w449
        n314 = Not(x=w449) -> (.not. x?=→"Laundry 1 Close":bool)
      }
      frame "04" {
        n315 = Type Cast(type=TRUE, x=w455) -> (*(type *) &x=w453:bool)
        "Laundry 2 Open" <- w453
        n316 = Not(x=w453) -> (.not. x?=→"Laundry 2 Close":bool)
      }
      frame "05" {
        n317 = Type Cast(type=TRUE, x=w459) -> (*(type *) &x=w457:bool)
        "Laundry 4 Open" <- w457
        n318 = Not(x=w457) -> (.not. x?=→"Laundry 4 Close":bool)
      }
      frame "06" {
        n319 = Type Cast(type=TRUE, x=w463) -> (*(type *) &x=w461:bool)
        "Bathroom 2 Open" <- w461
        n320 = Not(x=w461) -> (.not. x?=→"Bathroom 2 Close":bool)
      }
      frame "07" {
        n321 = Type Cast(type=TRUE, x=w467) -> (*(type *) &x=w465:bool)
        "Back Door  Open" <- w465
        n322 = Not(x=w465) -> (.not. x?=→"Back Door Close":bool)
      }
      frame "08" {
        n323 = Type Cast(type=TRUE, x=w471) -> (*(type *) &x=w469:bool)
        n324 = Not(x=w469) -> (.not. x?=w468:bool)
        n325 = local write "Front Door Close"(w468) -> ()
        n326 = local write "Bedroom 1 Close"(w468) -> ()
        n327 = local write "Bedroom 2 Close"(w468) -> ()
        n328 = local write "Laundry 1 Close"(w468) -> ()
        n329 = local write "Bedroom 1 Open"(w469) -> ()
        n330 = local write "Front Door Open"(w469) -> ()
        n331 = local write "Bedroom 2 Open"(w469) -> ()
        n332 = local write "Laundry 1 Open"(w469) -> ()
        n333 = local write "Laundry 2 Open"(w469) -> ()
        n334 = local write "Laundry 4 Open"(w469) -> ()
        n335 = local write "Back Door  Open"(w469) -> ()
        n336 = local write "Bathroom 2 Open"(w469) -> ()
        n337 = local write "Laundry 2 Close"(w468) -> ()
        n338 = local write "Laundry 4 Close"(w468) -> ()
        n339 = local write "Bathroom 2 Close"(w468) -> ()
        n340 = local write "Back Door Close"(w468) -> ()
      }
      frame "09" {
        n341 = Type Cast(type=TRUE, x=w474) -> (*(type *) &x=w472:bool)
        n342 = local write "Automation"(w472) -> ()
      }
    }
  }
  n343 = while {
    tunnel: w17 -> [w489]
    tunnel: w16 -> [w488]
    tunnel: [w480] -> w15
    tunnel: [w479] -> w14
    stop <- FALSE stop-if-true
    n344 = TCP Read "TCP Read for\nReceiving the\nData/Payload"(connection ID=w489, bytes to read=4, error in (no error)=w488) -> (connection ID out=w487:refnum<k5>, data out=w477:string, error out=w486:errorcluster)  [unwired: 2 in]
    n345 = Type Cast(type=65516, x=w477) -> (*(type *) &x=w476:i32)
    n346 = TCP Read "TCP Read for\nReceiving the\nString Length"(connection ID=w487, bytes to read=w476, error in (no error)=w486) -> (connection ID out=w480:refnum<k5>, data out=w484:string, error out=w479:errorcluster)  [unwired: 2 in]
    n347 = Search/Split String "Search/Split \nString"(string=w484, offset (0)=2) -> (substring before match=w482:string, match + rest of string=w481:string)  [unwired: 1 in, 1 out]
    n348 = case shown="\"06\"" w482 {
      tunnel: w481 -> [_ w492 w495 w498 w501 w504 w507 w510 w513 w516 w519 w522]
      frame Default {
      }
      frame "00" {
        n349 = Decimal String To Number "Decimal String \nTo Number"(string=w492) -> (number=w490:i32)  [unwired: 2 in, 1 out]
        n350 = To Unsigned Byte Integer "To Unsigned\n Byte Integer"(number=w490) -> (unsigned 8bit integer=w491:u8)
        n351 = local write "LivingRoomBrightness"(w491) -> ()
      }
      frame "01" {
        n352 = Decimal String To Number "Decimal String \nTo Number"(string=w495) -> (number=w494:i32)  [unwired: 2 in, 1 out]
        n353 = To Unsigned Byte Integer "To Unsigned\n Byte Integer"(number=w494) -> (unsigned 8bit integer=w493:u8)
        n354 = local write "Bedroom1Brightness"(w493) -> ()
      }
      frame "02" {
        n355 = Decimal String To Number "Decimal String \nTo Number"(string=w498) -> (number=w497:i32)  [unwired: 2 in, 1 out]
        n356 = To Unsigned Byte Integer "To Unsigned\n Byte Integer"(number=w497) -> (unsigned 8bit integer=w496:u8)
        n357 = local write "Bedroom2Brightness"(w496) -> ()
      }
      frame "03" {
        n358 = Decimal String To Number "Decimal String \nTo Number"(string=w501) -> (number=w500:i32)  [unwired: 2 in, 1 out]
        n359 = To Unsigned Byte Integer "To Unsigned\n Byte Integer"(number=w500) -> (unsigned 8bit integer=w499:u8)
        n360 = local write "Laundry1Brightness"(w499) -> ()
      }
      frame "04" {
        n361 = Decimal String To Number "Decimal String \nTo Number"(string=w504) -> (number=w503:i32)  [unwired: 2 in, 1 out]
        n362 = To Unsigned Byte Integer "To Unsigned\n Byte Integer"(number=w503) -> (unsigned 8bit integer=w502:u8)
        n363 = local write "Laundry2Brightness"(w502) -> ()
      }
      frame "05" {
        n364 = Decimal String To Number "Decimal String \nTo Number"(string=w507) -> (number=w506:i32)  [unwired: 2 in, 1 out]
        n365 = To Unsigned Byte Integer "To Unsigned\n Byte Integer"(number=w506) -> (unsigned 8bit integer=w505:u8)
        n366 = local write "Laundry3Brightness"(w505) -> ()
      }
      frame "06" {
        n367 = Decimal String To Number "Decimal String \nTo Number"(string=w510) -> (number=w509:i32)  [unwired: 2 in, 1 out]
        n368 = To Unsigned Byte Integer "To Unsigned\n Byte Integer"(number=w509) -> (unsigned 8bit integer=w508:u8)
        n369 = local write "Laundry4Brightness"(w508) -> ()
      }
      frame "07" {
        n370 = Decimal String To Number "Decimal String \nTo Number"(string=w513) -> (number=w512:i32)  [unwired: 2 in, 1 out]
        n371 = To Unsigned Byte Integer "To Unsigned\n Byte Integer"(number=w512) -> (unsigned 8bit integer=w511:u8)
        n372 = local write "Bathroom1Brightness"(w511) -> ()
      }
      frame "08" {
        n373 = Decimal String To Number "Decimal String \nTo Number"(string=w516) -> (number=w515:i32)  [unwired: 2 in, 1 out]
        n374 = To Unsigned Byte Integer "To Unsigned\n Byte Integer"(number=w515) -> (unsigned 8bit integer=w514:u8)
        n375 = local write "Bathroom2Brightness"(w514) -> ()
      }
      frame "09" {
        n376 = Decimal String To Number "Decimal String \nTo Number"(string=w519) -> (number=w518:i32)  [unwired: 2 in, 1 out]
        n377 = To Unsigned Byte Integer "To Unsigned\n Byte Integer"(number=w518) -> (unsigned 8bit integer=w517:u8)
        n378 = local write "KitchenBrightness"(w517) -> ()
      }
      frame "10" {
        n379 = Decimal String To Number "Decimal String \nTo Number"(string=w522) -> (number=w521:i32)  [unwired: 2 in, 1 out]
        n380 = To Unsigned Byte Integer "To Unsigned\n Byte Integer"(number=w521) -> (unsigned 8bit integer=w520:u8)
        n381 = local write "DiningBrightness"(w520) -> ()
      }
    }
  }
  n382 = while {
    stop <- FALSE stop-if-true
    # "Between lower temp and upper temp, randomize the temperature value"
    n383 = Random Number (0-1)() -> (number: 0 to 1=w529:dbl)
    n384 = Subtract(x="Upper Temp", y="Lower Temp") -> (x-y=w527:dbl)
    n385 = Multiply(x=w529, y=w527) -> (x*y=w526:dbl)
    n386 = Add(x=w526, y="Lower Temp") -> (x+y=→"Temperature Fluctuations" →"Thermometer":dbl)
    n387 = Wait (ms)(milliseconds to wait=u32 1000) -> ()  [unwired: 1 out]
  }
  n388 = TCP Close Connection "TCP Close \nConnection"(connection ID=w57, error in (no error)=w56) -> (error out=w55:errorcluster)  [unwired: 1 in, 1 out]
  n389 = TCP Close Connection "TCP Close \nConnection"(connection ID=w41, error in (no error)=w40) -> (error out=w39:errorcluster)  [unwired: 1 in, 1 out]
  n390 = call <vilib>:"Clear Errors.vi"("error in (no error)"=w55) -> ()  [unwired: 5 in, 2 out]
  n391 = call <vilib>:"Clear Errors.vi"("error in (no error)"=w39) -> ()  [unwired: 5 in, 2 out]
  n392 = TCP Close Connection "TCP Close \nConnection"(connection ID=w33, error in (no error)=w32) -> (error out=w31:errorcluster)  [unwired: 1 in, 1 out]
  n393 = TCP Close Connection "TCP Close \nConnection"(connection ID=w15, error in (no error)=w14) -> (error out=w13:errorcluster)  [unwired: 1 in, 1 out]
  n394 = while {
    stop <- FALSE stop-if-true
    n395 = local read "Vacation"() -> (w532:bool)
    n396 = case shown="True" w532 {
      frame False {
      }
      frame True {
        n397 = flat-sequence {
          frame #0 {
            n398 = local write "Living Room"(TRUE ("Living Room")) -> ()
          }
          frame #1 {
            n399 = local write "Living Room"(FALSE ("Living Room")) -> ()
            n400 = local write "Bedroom 1"(TRUE ("Bedroom 1")) -> ()
            n401 = Wait (ms)(milliseconds to wait=u32 4000) -> ()  [unwired: 1 out]
          }
          frame #2 {
            n402 = local write "Bedroom 1"(FALSE ("Bedroom 1")) -> ()
            n403 = local write "Bedroom 2"(TRUE ("Bedroom 2")) -> ()
            n404 = Wait (ms)(milliseconds to wait=u32 4000) -> ()  [unwired: 1 out]
          }
          frame #3 {
            n405 = local write "Bedroom 2"(FALSE ("Bedroom 2")) -> ()
            n406 = local write "Laundry 1"(TRUE ("Laundry 1")) -> ()
            n407 = Wait (ms)(milliseconds to wait=u32 4000) -> ()  [unwired: 1 out]
          }
          frame #4 {
            n408 = local write "Laundry 2"(TRUE ("Laundry 2")) -> ()
            n409 = local write "Laundry 1"(FALSE ("Laundry 1")) -> ()
            n410 = Wait (ms)(milliseconds to wait=u32 4000) -> ()  [unwired: 1 out]
          }
          frame #5 {
            n411 = local write "Laundry 2"(FALSE ("Laundry 2")) -> ()
            n412 = local write "Laundry 3"(TRUE ("Laundry 3")) -> ()
            n413 = Wait (ms)(milliseconds to wait=u32 4000) -> ()  [unwired: 1 out]
          }
          frame #6 {
            n414 = local write "Laundry 3"(FALSE ("Laundry 3")) -> ()
            n415 = local write "Laundry 4"(TRUE ("Laundry 4")) -> ()
            n416 = Wait (ms)(milliseconds to wait=u32 4000) -> ()  [unwired: 1 out]
          }
          frame #7 {
            n417 = local write "Bathroom 1"(TRUE ("Bathroom 1")) -> ()
            n418 = local write "Laundry 4"(FALSE ("Laundry 4")) -> ()
            n419 = Wait (ms)(milliseconds to wait=u32 4000) -> ()  [unwired: 1 out]
          }
          frame #8 {
            n420 = local write "Bathroom 1"(FALSE ("Bathroom 1")) -> ()
            n421 = local write "Bathroom 2"(TRUE ("Bathroom 2")) -> ()
            n422 = Wait (ms)(milliseconds to wait=u32 4000) -> ()  [unwired: 1 out]
          }
          frame #9 {
            n423 = local write "Bathroom 2"(FALSE ("Bathroom 2")) -> ()
            n424 = local write "Kitchen"(TRUE ("Kitchen")) -> ()
            n425 = Wait (ms)(milliseconds to wait=u32 4000) -> ()  [unwired: 1 out]
          }
          frame #10 {
            n426 = local write "Kitchen"(FALSE ("Kitchen")) -> ()
            n427 = Wait (ms)(milliseconds to wait=u32 4000) -> ()  [unwired: 1 out]
            n428 = local write "Dining"(TRUE ("Dining")) -> ()
          }
        }
        n429 = local write "Living Room"(FALSE ("Living Room")) -> ()
        n430 = local write "Laundry 1"(FALSE ("Laundry 1")) -> ()
        n431 = local write "Laundry 2"(FALSE ("Laundry 2")) -> ()
        n432 = local write "Laundry 3"(FALSE ("Laundry 3")) -> ()
        n433 = local write "Laundry 4"(FALSE ("Laundry 4")) -> ()
        n434 = local write "Bathroom 1"(FALSE ("Bathroom 1")) -> ()
        n435 = local write "Bathroom 2"(FALSE ("Bathroom 2")) -> ()
        n436 = local write "Kitchen"(FALSE ("Kitchen")) -> ()
        n437 = local write "Dining"(FALSE ("Dining")) -> ()
      }
    }
  }
  n438 = call <vilib>:"Clear Errors.vi"("error in (no error)"=w31) -> ()  [unwired: 5 in, 2 out]
  n439 = call <vilib>:"Clear Errors.vi"("error in (no error)"=w13) -> ()  [unwired: 5 in, 2 out]
  n440 = while {
    stop <- FALSE stop-if-true
    n441 = local read "Automation"() -> (w574:bool)
    n442 = event shown="[9] \"Back Door Close\": Mouse Down" {
      selector: _ -> [_ _ _ _ _ _ _ _ _ _]
      dyn-events: _ -> [_ _ _ _ _ _ _ _ _ _]
      timeout: _ -> [_ _ _ _ _ _ _ _ _ _]
      tunnel: w574 -> [w575 w578 w581 w584 w587 w590 w593 w596 _ _]
      event "Front Door Close": Mouse Enter {
        n443 = event-data() -> ()  [unwired: 1 in, 4 out]
        n444 = case shown="True" w575 {
          frame False {
          }
          frame True {
            n445 = local write "Front Door Open"(TRUE ("Front Door Open")) -> ()
            n446 = local write "Front Door Close"(FALSE ("Front Door Close")) -> ()
          }
        }
      }
      event "Bedroom 1 Close": Mouse Enter {
        n447 = event-data() -> ()  [unwired: 1 in, 4 out]
        n448 = case shown="True" w578 {
          frame False {
          }
          frame True {
            n449 = local write "Bedroom 1 Open"(TRUE ("Bedroom 1 Open")) -> ()
            n450 = local write "Bedroom 1 Close"(FALSE ("Bedroom 1 Close")) -> ()
          }
        }
      }
      event "Bedroom 2 Close": Mouse Enter {
        n451 = event-data() -> ()  [unwired: 1 in, 4 out]
        n452 = case shown="True" w581 {
          frame False {
          }
          frame True {
            n453 = local write "Bedroom 2 Close"(FALSE ("Bedroom 2 Close")) -> ()
            n454 = local write "Bedroom 2 Open"(TRUE ("Bedroom 2 Open")) -> ()
          }
        }
      }
      event "Laundry 1 Close": Mouse Enter {
        n455 = event-data() -> ()  [unwired: 1 in, 4 out]
        n456 = case shown="True" w584 {
          frame False {
          }
          frame True {
            n457 = local write "Laundry 1 Open"(TRUE ("Laundry 1 Open")) -> ()
            n458 = local write "Laundry 1 Close"(FALSE ("Laundry 1 Close")) -> ()
          }
        }
      }
      event "Laundry 2 Close": Mouse Enter {
        n459 = event-data() -> ()  [unwired: 1 in, 4 out]
        n460 = case shown="True" w587 {
          frame False {
          }
          frame True {
            n461 = local write "Laundry 2 Open"(TRUE ("Laundry 1 Open")) -> ()
            n462 = local write "Laundry 2 Close"(FALSE ("Laundry 1 Close")) -> ()
          }
        }
      }
      event "Laundry 4 Close": Mouse Enter {
        n463 = event-data() -> ()  [unwired: 1 in, 4 out]
        n464 = case shown="True" w590 {
          frame False {
          }
          frame True {
            n465 = local write "Laundry 4 Close"(FALSE ("Laundry 4 Close")) -> ()
            n466 = local write "Laundry 4 Open"(TRUE ("Laundry 4 Open")) -> ()
          }
        }
      }
      event "Bathroom 2 Close": Mouse Enter {
        n467 = event-data() -> ()  [unwired: 1 in, 4 out]
        n468 = case shown="True" w593 {
          frame False {
          }
          frame True {
            n469 = local write "Bathroom 2 Open"(TRUE ("Laundry 4 Open")) -> ()
            n470 = local write "Bathroom 2 Close"(FALSE ("Laundry 4 Close")) -> ()
          }
        }
      }
      event "Back Door Close": Mouse Enter {
        n471 = event-data() -> ()  [unwired: 1 in, 4 out]
        n472 = case shown="True" w596 {
          frame False {
          }
          frame True {
            n473 = local write "Back Door Close"(FALSE ("Laundry 4 Close")) -> ()
            n474 = local write "Back Door  Open"(TRUE ("Laundry 4 Open")) -> ()
          }
        }
      }
      event "Front Door Close": Mouse Down {
        n475 = event-data() -> ("Mods.Double Click"=w601:bool)  [unwired: 1 in]
        n476 = local read "Front Door Close"() -> (w599:bool)
        n477 = And(x=w599, y=w601) -> (x .and. y?=w600:bool)
        n478 = case shown="True" w600 {
          frame False {
          }
          frame True {
            n479 = call <vilib>:"Beep.vi"("use system alert? (T)"=TRUE) -> ()  [unwired: 11 in]
          }
        }
      }
      event "Back Door Close": Mouse Down {
        n480 = event-data() -> ("Mods.Double Click"=w605:bool)  [unwired: 1 in]
        n481 = local read "Back Door Close"() -> (w603:bool)
        n482 = And(x=w603, y=w605) -> (x .and. y?=w604:bool)
        n483 = case shown="True" w604 {
          frame False {
          }
          frame True {
            n484 = call <vilib>:"Beep.vi"("use system alert? (T)"=TRUE) -> ()  [unwired: 11 in]
          }
        }
      }
    }
  }
  n485 = call <vilib>:"TCP Listen.vi"("timeout ms (wait forever: -1)"=-1, "port"=u16 54000, "service name"="localhost") -> ("error out"=w51:errorcluster, "connection ID"=w50:refnum<k5>)  [unwired: 4 in, 3 out]
  n486 = while {
    tunnel: w50 -> [w620]
    tunnel: w51 -> [w619]
    tunnel: [w615] -> w52
    tunnel: [w614] -> w53
    tunnel: ["TV"] -> w1
    stop <- FALSE stop-if-true
    n487 = TCP Read "TCP Read for\nReceiving the\nData/Payload"(connection ID=w620, bytes to read=4, error in (no error)=w619) -> (connection ID out=w618:refnum<k5>, data out=w612:string, error out=w617:errorcluster)  [unwired: 2 in]
    n488 = Type Cast(type=0, x=w612) -> (*(type *) &x=w611:i32)
    n489 = Automation Open "Automation \nOpen"(Automation Refnum="TV") -> (Automation Refnum=w608:refnum<k7>)  [unwired: 3 in, 1 out]
    n490 = TCP Read "TCP Read for\nReceiving the\nString Length"(connection ID=w618, bytes to read=w611, error in (no error)=w617) -> (connection ID out=w615:refnum<k5>, data out=w609:string, error out=w614:errorcluster)  [unwired: 2 in]
    n491 = case shown="\"10\"" w609 {
      tunnel: w608 -> [w621 w622 w629 w635 w637 w640 w643 w648 w649 w655 w660 w665]
      frame Default {
        n492 = Close Reference(reference=w621) -> ()  [unwired: 1 in, 1 out]
      }
      frame "00" {
        n493 = Close Reference(reference=w622) -> ()  [unwired: 1 in, 1 out]
        n494 = property on="TV" class="AXCont"() -> ("Visible"=w624:bool)  [unwired: 2 in, 2 out]
        n495 = Not(x=w624) -> (.not. x?=w623:bool)
        n496 = property on="TV" class="AXCont"("Visible"=w623) -> ()  [unwired: 2 in, 2 out]
      }
      frame "01" {
        n497 = call <vilib>:"Application Directory.vi"() -> ("Application Directory"=w628:path)
        n498 = Build Path(base path=w628, name or relative path=path "ch1.mp4") -> (appended path=w626:path)
        n499 = Path To String(path=w626) -> (string=w625:string)
        n500 = property on="Property Node" class="IWMPPlayer4"(reference=w629, "URL"=w625) -> (reference out=w630:refnum<k7>)  [unwired: 1 in, 1 out]
        n501 = Close Reference(reference=w630) -> ()  [unwired: 1 in, 1 out]
      }
      frame "02" {
        n502 = call <vilib>:"Application Directory.vi"() -> ("Application Directory"=w634:path)
        n503 = Build Path(base path=w634, name or relative path=path "ch2.mp4") -> (appended path=w632:path)
        n504 = Path To String(path=w632) -> (string=w631:string)
        n505 = property class="IWMPPlayer4"(reference=w635, "URL"=w631) -> (reference out=w636:refnum<k7>)  [unwired: 1 in, 1 out]
        n506 = Close Reference(reference=w636) -> ()  [unwired: 1 in, 1 out]
      }
      frame "03" {
        n507 = property class="IWMPPlayer4"(reference=w637) -> ("controls"=w638:refnum<k7>)  [unwired: 1 in, 2 out]
        n508 = invoke class="IWMPControls" method="play"(reference=w638) -> (reference out=w639:refnum<k7>)  [unwired: 2 in, 2 out]
        n509 = Close Reference(reference=w639) -> ()  [unwired: 1 in, 1 out]
      }
      frame "04" {
        n510 = property class="IWMPPlayer4"(reference=w640) -> ("controls"=w641:refnum<k7>)  [unwired: 1 in, 2 out]
        n511 = invoke class="IWMPControls" method="pause"(reference=w641) -> (reference out=w642:refnum<k7>)  [unwired: 2 in, 2 out]
        n512 = Close Reference(reference=w642) -> ()  [unwired: 1 in, 1 out]
      }
      frame "05" {
        n513 = property class="IWMPPlayer4"(reference=w643) -> ("controls"=w644:refnum<k7>)  [unwired: 1 in, 2 out]
        n514 = invoke class="IWMPControls" method="stop"(reference=w644) -> (reference out=w645:refnum<k7>)  [unwired: 2 in, 2 out]
        n515 = Close Reference(reference=w645) -> ()  [unwired: 1 in, 1 out]
      }
      frame "06" {
        n516 = property class="IWMPPlayer4"(reference=w648) -> ("controls"=w647:refnum<k7>)  [unwired: 1 in, 2 out]
        n517 = invoke class="IWMPControls" method="fastReverse"(reference=w647) -> (reference out=w646:refnum<k7>)  [unwired: 2 in, 2 out]
        n518 = Close Reference(reference=w646) -> ()  [unwired: 1 in, 1 out]
      }
      frame "07" {
        n519 = property class="IWMPPlayer4"(reference=w649) -> ("controls"=w650:refnum<k7>)  [unwired: 1 in, 2 out]
        n520 = invoke class="IWMPControls" method="fastForward"(reference=w650) -> (reference out=w651:refnum<k7>)  [unwired: 2 in, 2 out]
        n521 = Close Reference(reference=w651) -> ()  [unwired: 1 in, 1 out]
      }
      frame "10" {
        n522 = property class="IWMPPlayer4"(reference=w655) -> ("settings"=w654:refnum<k7>)  [unwired: 1 in, 2 out]
        n523 = property class="IWMPSettings"(reference=w654) -> ("volume"=w653:i32)  [unwired: 1 in, 2 out]
        n524 = Decrement(x=w653) -> (x-1=w652:i32)
        n525 = property class="IWMPSettings"(reference=w654, "volume"=w652) -> (reference out=w656:refnum<k7>)  [unwired: 1 in, 1 out]
        n526 = Close Reference(reference=w656) -> ()  [unwired: 1 in, 1 out]
      }
      frame "11" {
        n527 = property class="IWMPPlayer4"(reference=w660) -> ("settings"=w659:refnum<k7>)  [unwired: 1 in, 2 out]
        n528 = property class="IWMPSettings"(reference=w659) -> ("volume"=w658:i32)  [unwired: 1 in, 2 out]
        n529 = Increment(x=w658) -> (x+1=w657:i32)
        n530 = property class="IWMPSettings"(reference=w659, "volume"=w657) -> (reference out=w661:refnum<k7>)  [unwired: 1 in, 1 out]
        n531 = Close Reference(reference=w661) -> ()  [unwired: 1 in, 1 out]
      }
      frame "12" {
        n532 = property class="IWMPPlayer4"(reference=w665) -> ("settings"=w664:refnum<k7>)  [unwired: 1 in, 2 out]
        n533 = property class="IWMPSettings"(reference=w664) -> ("mute"=w663:bool)  [unwired: 1 in, 2 out]
        n534 = Not(x=w663) -> (.not. x?=w662:bool)
        n535 = property class="IWMPSettings"(reference=w664, "mute"=w662) -> (reference out=w666:refnum<k7>)  [unwired: 1 in, 1 out]
        n536 = Close Reference(reference=w666) -> ()  [unwired: 1 in, 1 out]
      }
    }
  }
  n537 = while {
    tunnel: w1 -> [w667]
    stop <- FALSE stop-if-true
    w669 = 21 ("y")
    n538 = Get Date/Time In Seconds() -> (seconds since 1Jan1904=w680:timestamp)
    n539 = Seconds To Date/Time(time stamp (now)=w680) -> (date time rec=w679:T1)  [unwired: 1 in]
    n540 = local read "NightTV"() -> (w674:bool)
    n541 = Unbundle By Name "Unbundle By Name"(w679) -> ("hour"=w670:i32)
    n542 = Not(x=w674) -> (.not. x?=w673:bool)
    n543 = Greater Or Equal?(x=w670, y=w669) -> (x >= y?=w676:bool)
    n544 = Less?(x=w670, y=7) -> (x < y?=w675:bool)
    n545 = Equal?(x=w670, y=w669) -> (x = y?=w668:bool)
    n546 = Or(x=w676, y=w675) -> (x .or. y?=w672:bool)
    n547 = And(x=w672, y=w673) -> (x .and. y?=w671:bool)
    n548 = case shown="True" w671 {
      tunnel: w667 -> [_ w682]
      frame False {
      }
      frame True {
        n549 = local write "NightTV"(TRUE ("NightTV")) -> ()
        n550 = Automation Open "Automation \nOpen"(Automation Refnum=w682) -> (Automation Refnum=w686:refnum<k7>)  [unwired: 3 in, 1 out]
        n551 = property class="IWMPPlayer4"(reference=w686) -> ("settings"=w687:refnum<k7>)  [unwired: 1 in, 2 out]
        n552 = property class="IWMPSettings"(reference=w687, "volume"=20) -> (reference out=w684:refnum<k7>)  [unwired: 1 in, 1 out]
        n553 = Close Reference(reference=w684) -> ()  [unwired: 1 in, 1 out]
      }
    }
    n554 = case shown="False" w668 {
      frame False {
      }
      frame True {
        n555 = local write "NightTV"(FALSE ("NightTV")) -> ()
      }
    }
  }
  n556 = while {
    stop <- FALSE stop-if-true
    n557 = Get Date/Time In Seconds() -> (seconds since 1Jan1904=w696:timestamp)
    n558 = Seconds To Date/Time "Seconds To \nDate/Time"(time stamp (now)=w696) -> (date time rec=w695:T1)  [unwired: 1 in]
    n559 = Unbundle By Name "Unbundle By Name"(w695) -> ("hour"=w692:i32)
    n560 = Greater Or Equal?(x=w692, y=9) -> (x >= y?=w690:bool)
    n561 = Less?(x=w692, y=19) -> (x < y?=w689:bool)
    n562 = And(x=w690, y=w689) -> (x .and. y?=w688:bool)
    n563 = case shown="True" w688 {
      frame False {
        n564 = local read "DayCurtain"() -> (w697:bool)
        n565 = case shown="True" w697 {
          frame False {
          }
          frame True {
            n566 = local write "Bedroom 1"(1.0 ("Bedroom 1")) -> ()
            n567 = local write "Bedroom 2"(1.0 ("Bedroom 2")) -> ()
            n568 = local write "DayCurtain"(FALSE ("NightTV")) -> ()
          }
        }
      }
      frame True {
        n569 = local read "DayCurtain"() -> (w701:bool)
        n570 = case shown="True" w701 {
          frame False {
            n571 = local write "Bedroom 1"(0.0 ("Bedroom 1")) -> ()
            n572 = local write "Bedroom 2"(0.0 ("Bedroom 2")) -> ()
            n573 = local write "DayCurtain"(TRUE ("NightTV")) -> ()
          }
          frame True {
          }
        }
      }
    }
  }
  n574 = Get Date/Time In Seconds() -> (seconds since 1Jan1904=w23:timestamp)
  n575 = Seconds To Date/Time "Seconds To \nDate/Time"(time stamp (now)=w23) -> (date time rec=w24:T1)  [unwired: 1 in]
  n576 = Unbundle By Name "Unbundle By Name"(w24) -> ("hour"=w26:i32)
  n577 = Greater Or Equal?(x=w26, y=9) -> (x >= y?=w28:bool)
  n578 = Less?(x=w26, y=19) -> (x < y?=w29:bool)
  n579 = And(x=w28, y=w29) -> (x .and. y?=w22:bool)
  n580 = Not(x=w22) -> (.not. x?=→"DayCurtain":bool)
  n581 = TCP Close Connection "TCP Close \nConnection"(connection ID=w52, error in (no error)=w53) -> (error out=w54:errorcluster)  [unwired: 1 in, 1 out]
  n582 = call <vilib>:"Clear Errors.vi"("error in (no error)"=w54) -> ()  [unwired: 5 in, 2 out]
  "NightTV" <- FALSE
  "LivingRoomBrightness" <- w3
  "Bedroom1Brightness" <- w3
  "Laundry1Brightness" <- w3
  "Laundry2Brightness" <- w3
  "Laundry3Brightness" <- w3
  "Laundry4Brightness" <- w3
  "Bathroom1Brightness" <- w3
  "Bathroom2Brightness" <- w3
  "KitchenBrightness" <- w3
  "DiningBrightness" <- w3
  "Bedroom2Brightness" <- w3
  "Vacation" <- FALSE ("Vacation")
  "Automation" <- FALSE ("Automation")
